vi "SaveMeasurementDataToFileSubVI.vi"(0 "VISA Refnum in":refnum<visa-resource-name>, 1 "Array of Measurement":T1(array[cluster]), 2 "Output Directory":path, 3 "Object number":string, 4 "Array of Time for Measurement":string[](array[string]), 5 "error in (no error)":errorcluster, 7 "NDI Tool":string) -> (6 "VISA Refnum out":refnum<visa-resource-name>, 8 "error out":errorcluster)   [LabVIEW 2013]
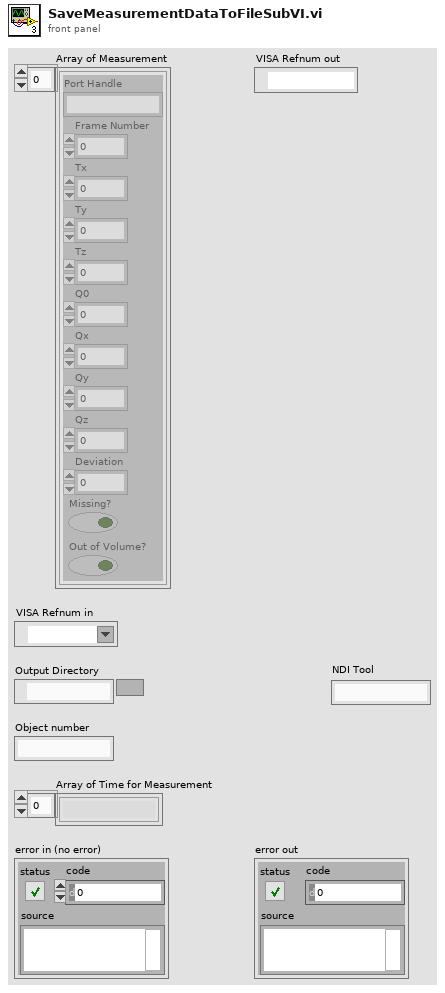
[diagram p1: front panel]
types:
  T1 = cluster{"Port Handle":string, "Frame Number":u32, "Tx":dbl, "Ty":dbl, "Tz":dbl, "Q0":dbl, "Qx":dbl, "Qy":dbl, "Qz":dbl, "Deviation":dbl, "Missing?":bool, "Out of Volume?":bool}[]
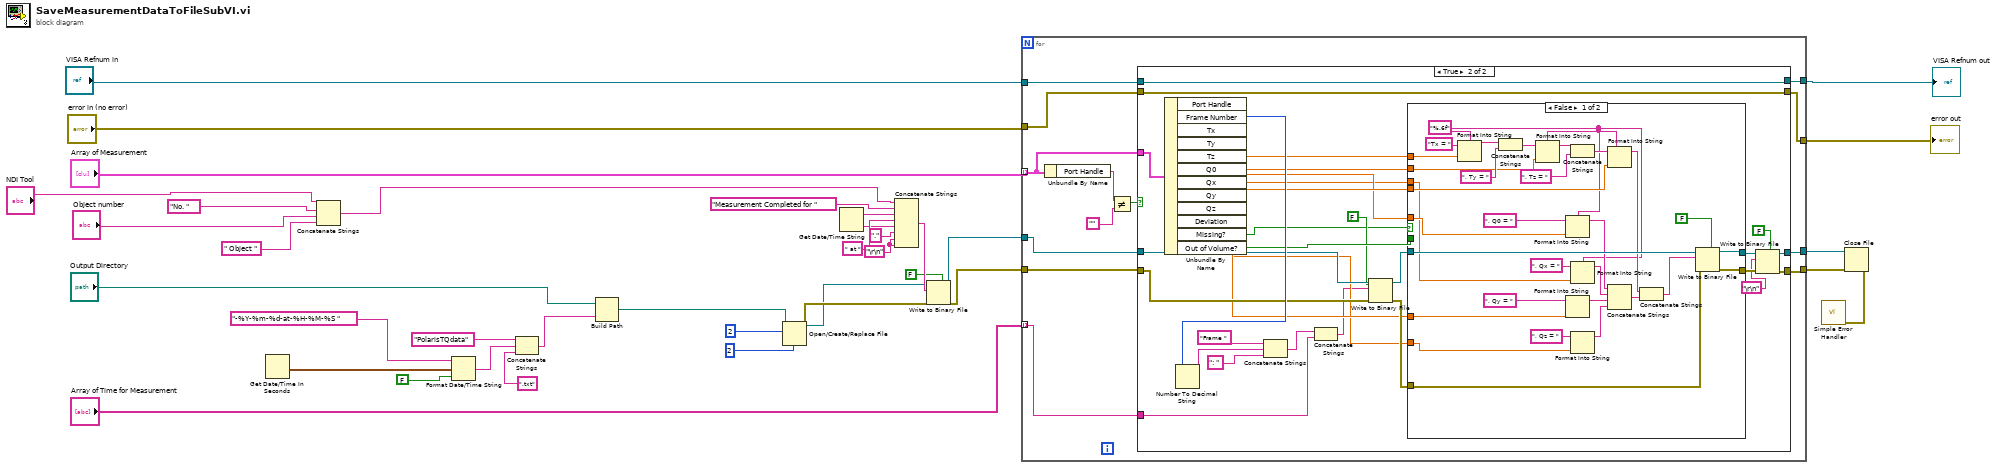
[diagram p0: block diagram]
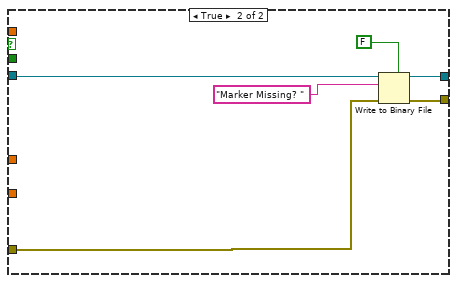
[diagram p3: hidden frame]
diagram:
  w28 = "\r\n"
  n1 = Get Date/Time In Seconds() -> (seconds since 1Jan1904=w20:timestamp)
  n2 = Concatenate Strings("NDI Tool", "No. ", "Object number", " Object ") -> (w6:string)
  n3 = Format Date/Time String(time format string (%c)="-%Y-%m-%d-at-%H-%M-%S ", seconds (now)=w20, UTC format=FALSE) -> (date/time string=w23:string)
  n4 = Concatenate Strings("PolarisTQdata", w23, ".txt") -> (w22:string)
  n5 = Build Path(base path="Output Directory", name or relative path=w22) -> (appended path=w21:path)
  n6 = Open/Create/Replace File(file path (use dialog)=w21, operation (0:open)=i8 2, access (0:read/write)=i8 2) -> (refnum out=w13:refnum<file>, error out=w14:errorcluster)  [unwired: 3 in, 1 out]
  n7 = Get Date/Time String() -> (date string=w33:string, time string=w31:string)  [unwired: 3 in]
  n8 = Concatenate Strings(w6, "Measurement Completed for ", w33, " at ", w31, "." ("string"), w28, w28) -> (w30:string)
  n9 = Write to Binary File(file (use dialog)=w13, data=w30, error in=w14, 5:FALSE ("prepend array or string size? (T)")) -> (refnum out=w11:refnum<file>, error out=w12:errorcluster)  [unwired: 2 in, 1 out]
  n10 = for {
    tunnel: w11 -> [w50]
    tunnel: [w48] -> w9
    tunnel: "Array of Measurement" -> [w42] mode=indexing
    tunnel: "Array of Time for Measurement" -> [w43] mode=indexing
    tunnel: "VISA Refnum in" -> [w41]
    tunnel: "error in (no error)" -> [w38]
    tunnel: [w40] -> w7
    tunnel: [w39] -> w2
    tunnel: w12 -> [w49]
    tunnel: [w47] -> w10
    n11 = Unbundle By Name(w42) -> ("Port Handle"=w46:string)
    n12 = Not Equal?(x=w46, y="") -> (x != y?=w45:bool)
    n13 = case shown="True" w45 {
      tunnel: w50 -> [w54 w83]
      tunnel: w49 -> [w53 w82]
      tunnel: [w54 w75] -> w48
      tunnel: [w53 w74] -> w47
      tunnel: w43 -> [_ w60]
      tunnel: w42 -> [_ w63]
      tunnel: w41 -> [w52 w57]
      tunnel: w38 -> [w51 w56]
      tunnel: [w52 w57] -> w40
      tunnel: [w51 w56] -> w39
      frame False {
      }
      frame True {
        n14 = Unbundle By Name(w63) -> ("Frame Number"=w84:u32, "Tx"=w79:dbl, "Ty"=w78:dbl, "Tz"=w77:dbl, "Q0"=w70:dbl, "Qx"=w69:dbl, "Qy"=w68:dbl, "Qz"=w67:dbl, "Missing?"=w55:bool, "Out of Volume?"=w73:bool)  [unwired: 2 out]
        n15 = Number To Decimal String(number=w84) -> (decimal integer string=w65:string)  [unwired: 1 in]
        n16 = Concatenate Strings("Frame ", w65, ": " ("string")) -> (w61:string)
        n17 = Concatenate Strings(w61, w60) -> (w62:string)
        n18 = Write to Binary File(file (use dialog)=w83, data=w62, error in=w82, 5:FALSE ("prepend array or string size? (T)")) -> (refnum out=w81:refnum<file>, error out=w80:errorcluster)  [unwired: 2 in, 1 out]
        n19 = case shown="False" w55 {
          tunnel: w81 -> [w104 w117]
          tunnel: w80 -> [w103 w118]
          tunnel: [w105 w121] -> w76
          tunnel: w79 -> [w114 _]
          tunnel: w78 -> [w110 _]
          tunnel: w77 -> [w106 _]
          tunnel: w73 -> [_ _]
          tunnel: w70 -> [w100 _]
          tunnel: w69 -> [w93 _]
          tunnel: w68 -> [w88 _]
          tunnel: w67 -> [w87 _]
          tunnel: [w85 w120] -> w58
          frame False {
            w95 = "%.6f" ("format string")
            n20 = Format Into String(format string=w95, initial string="Tx = ", w114) -> (resulting string=w113:string)  [unwired: 1 in, 1 out]
            n21 = Concatenate Strings(w113, ", Ty = ") -> (w111:string)
            n22 = Format Into String(format string=w95, initial string=w111, w110) -> (resulting string=w109:string)  [unwired: 1 in, 1 out]
            n23 = Format Into String(format string=w95, initial string=", Q0 = ", w100) -> (resulting string=w97:string)  [unwired: 1 in, 1 out]
            n24 = Format Into String(initial string=", Qy = ", w88) -> (resulting string=w92:string)  [unwired: 2 in, 1 out]
            n25 = Concatenate Strings(w109, ", Tz = ") -> (w108:string)
            n26 = Format Into String(format string=w95, initial string=", Qx = ", w93) -> (resulting string=w94:string)  [unwired: 1 in, 1 out]
            n27 = Format Into String(initial string=", Qz = ", w87) -> (resulting string=w91:string)  [unwired: 2 in, 1 out]
            n28 = Format Into String(format string=w95, initial string=w108, w106) -> (resulting string=w102:string)  [unwired: 1 in, 1 out]
            n29 = Concatenate Strings(w97, w94, w92, w91) -> (w98:string)
            n30 = Concatenate Strings(w102, w98) -> (w86:string)
            n31 = Write to Binary File(file (use dialog)=w104, data=w86, error in=w103, 5:FALSE ("prepend array or string size? (T)")) -> (refnum out=w85:refnum<file>, error out=w105:errorcluster)  [unwired: 2 in, 1 out]
          }
          frame True {
            n32 = Write to Binary File(file (use dialog)=w117, data="Marker Missing? ", error in=w118, 5:FALSE ("prepend array or string size? (T)")) -> (refnum out=w120:refnum<file>, error out=w121:errorcluster)  [unwired: 2 in, 1 out]
          }
        }
        n33 = Write to Binary File(file (use dialog)=w58, data="\r\n", error in=w76, 5:FALSE ("prepend array or string size? (T)")) -> (refnum out=w75:refnum<file>, error out=w74:errorcluster)  [unwired: 2 in, 1 out]
      }
    }
  }
  "VISA Refnum out" <- w7
  "error out" <- w2
  n34 = Close File(refnum=w9, error in=w10) -> (error out=w27:errorcluster)  [unwired: 1 out]
  n35 = call <vilib>:"Simple Error Handler.vi"("error in (no error)"=w27) -> ()  [unwired: 4 in, 5 out]
